vi "Log.vi"(6 "originVI":string, 7 "sourceTag":string, 8 "error in (no error)":errorcluster, 9 "message":string, 10 "level":T1=enum."INFO", 11 "Logger in":refnum<class "Logger.lvclass">) -> (0 "error out":errorcluster, 3 "Logger out":refnum<class "Logger.lvclass">)   [LabVIEW 2026, in "Lumberjack.lvlib" / "Logger.lvclass"]
doc: "Logs a message at the given severity through the resolved logger.\nBuilds a Statement (severity, message, sourceTag/origin) and enqueues it to every appender in the current Snapshot for asynchronous handling; the global threshold gates emission (stage 1) and each appender re-gates on its own threshold and filter (stage 2). No-op passthrough if no logger resolves.\nLumberjack.lvlib, Logger.lvclass, public; the hot-path entry that Info/Warn/Error/Fatal/Debug/Trace wrap."
uses:
  Logger.lvclass
  TypeDefs/Severity.ctl
  Logger.lvclass/Logger.ctl
  TypeDefs/Statement.ctl
  Lumberjack.lvlib
  Core/Messages/LogStatementMsg.lvclass/LogStatementMsg.lvclass
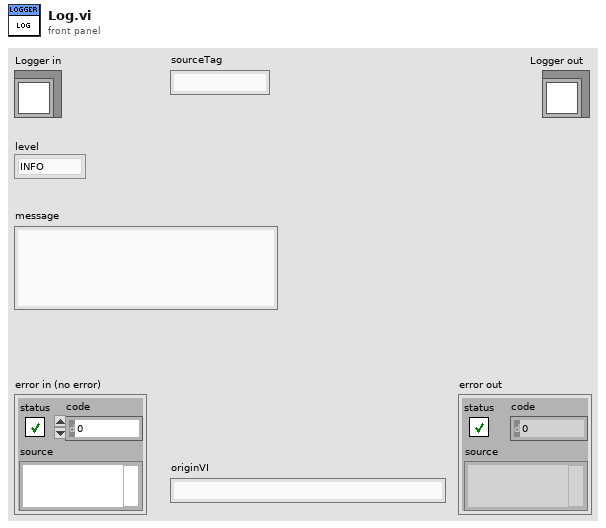
[diagram p1: front panel]
types:
  T1 = typedef "Lumberjack.lvlib/Severity.ctl" = enum16{"OFF", "FATAL", "ERROR", "WARN", "INFO", "DEBUG", "TRACE", "ALL"}
  T2 = typedef "Lumberjack.lvlib/Snapshot.ctl" = cluster{"globalThreshold":T1, "appenders":cluster{"id":string, "enqueuer":refnum<class "Message Enqueuer.lvclass">}[]}
  T3 = cluster{"id":string, "enqueuer":refnum<class "Message Enqueuer.lvclass">}[]
  T4 = typedef "Lumberjack.lvlib/Statement.ctl" = cluster{"timestamp":timestamp, "level":T1, "sourceTag":string, "originVI":string, "message":string}
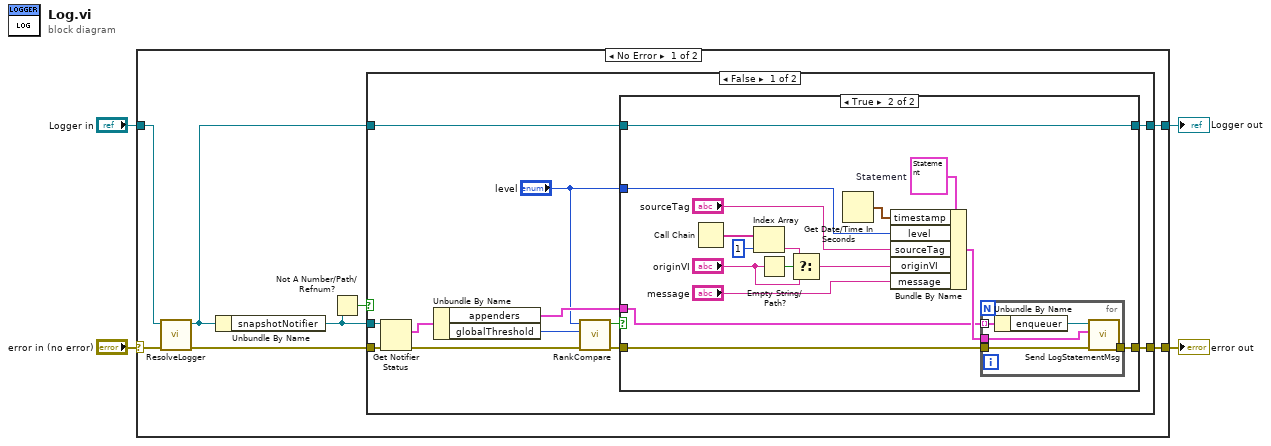
[diagram p0: block diagram]
diagram:
  n1 = case shown="No Error" "error in (no error)" {
    selector: "error in (no error)" -> [w10 w50]
    tunnel: [w12 w50] -> w4
    tunnel: "Logger in" -> [w11 w51]
    tunnel: [w6 w51] -> w1
    frame No Error {
      n2 = call "ResolveLogger.vi"("error in (no error)"=w10, "Logger in"=w11) -> ("error out"=w8:errorcluster, "Logger out"=w7:refnum<class "Logger.lvclass">)  [unwired: 8 in]
      n3 = Unbundle By Name(w7) -> ("snapshotNotifier"=w5:refnum<notifier>)
      n4 = Not A Number/Path/Refnum?(number/path/refnum=w5) -> (NaN/Path/Refnum?=w9:bool)
      n5 = case shown="False" w9 {
        tunnel: [w16 w49] -> w12
        tunnel: w8 -> [w24 w49]
        tunnel: w7 -> [w18 w48]
        tunnel: [w17 w48] -> w6
        tunnel: w5 -> [w23 _]
        frame False {
          n6 = Get Notifier Status(notifier=w23, error in (no error)=w24) -> (current notification=w22:T2, error out=w20:errorcluster)  [unwired: 3 out]
          n7 = Unbundle By Name(w22) -> ("appenders"=w14:T3, "globalThreshold"=w21:T1)
          n8 = call "RankCompare.vi"("error in (no error)"=w20, "Threshold"=w21, "Level"="level") -> ("error out"=w19:errorcluster, "Passes"=w15:bool)  [unwired: 7 in]
          n9 = case shown="True" w15 {
            tunnel: w19 -> [w26 w30]
            tunnel: w18 -> [w25 w42]
            tunnel: [w25 w42] -> w17
            tunnel: [w26 w29] -> w16
            tunnel: w14 -> [_ w27]
            tunnel: "level" -> [_ w31]
            frame False {
            }
            frame True {
              w36 = T4 {"timestamp"=timestamp(0 s since 1904-01-01), "level"=enum."INFO", "sourceTag"="", "originVI"="", "message"=""}  # Statement
              n10 = Call Chain() -> (call chain=w41:string[])
              n11 = Index Array(array=w41, index=1) -> (element=w37:string)
              n12 = Empty String/Path?(string/path="originVI") -> (empty?=w38:bool)
              n13 = Select(t=w37, s=w38, f="originVI") -> (s? t:f=w32:string)
              n14 = Get Date/Time In Seconds() -> (seconds since 1Jan1904=w35:timestamp)
              n15 = Bundle By Name(cluster=w36, "timestamp"=w35, "level"=w31, "sourceTag"="sourceTag", "originVI"=w32, "message"="message") -> (w28:T4)
              n16 = for {
                tunnel: w30 -> [w47]
                tunnel: [w46] -> w29
                tunnel: w27 -> [w44] mode=indexing
                tunnel: w28 -> [w45]
                n17 = Unbundle By Name(w44) -> ("enqueuer"=w43:refnum<class "Message Enqueuer.lvclass">)
                n18 = call "Send LogStatementMsg.vi"("error in (no error)"=w47, "Statement"=w45, "Enqueuer in"=w43) -> ("error out"=w46:errorcluster)  [unwired: 7 in, 1 out]
              }
            }
          }
        }
        frame True {
        }
      }
    }
    frame Error {
    }
  }
  "Logger out" <- w1
  "error out" <- w4
